vi "SADD.vi"(0 "TCP session out":refnum<k5>, 1 "Key":string, 5 "Members":string[](array[string]), 11 "error in":errorcluster) -> (4 "TCP session out":refnum<k5>, 6 "Data":T1, 15 "error out":errorcluster)   [LabVIEW 2023]
uses:
  SubVIs/Controls/redis-data.ctl
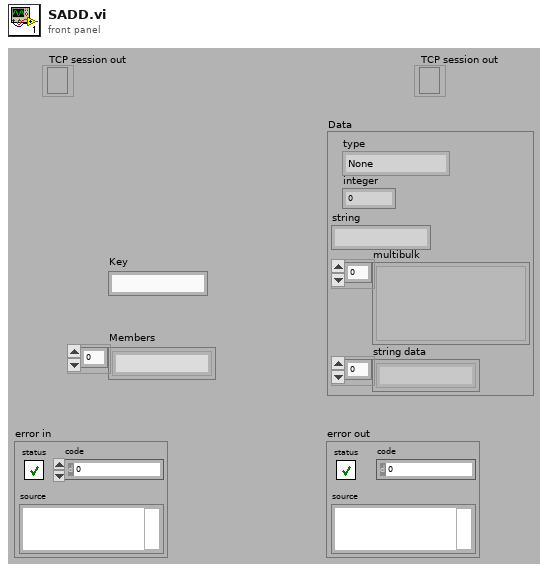
[diagram p1: front panel]
types:
  T1 = typedef "redis-data.ctl" = cluster{"type":enum16{"None", "Error", "Status", "Nil", "Integer", "String", "Multibulk"}, "integer":i64, "string":string, "multibulk":variant[], "string data":string[]}
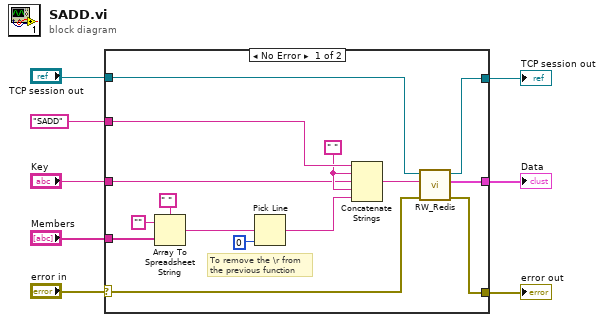
[diagram p0: block diagram]
diagram:
  n1 = case shown="No Error" "error in" {
    selector: "error in" -> [w21 w25]
    tunnel: "Members" -> [w14 _]
    tunnel: "SADD" -> [w23 _]
    tunnel: "TCP session out" -> [w10 w24]
    tunnel: [w20 w25] -> w6
    tunnel: [w19 _] -> w3
    tunnel: "Key" -> [w11 _]
    tunnel: [w9 w24] -> w1
    frame No Error {
      w13 = " "
      # "To remove the \\r from\nthe previous function"
      n2 = Array To Spreadsheet String(delimiter (Tab)=" ", array=w14, 3:"" ("format string")) -> (spreadsheet string=w17:string)
      n3 = Pick Line(multi-line string=w17, line index=0) -> (output string=w12:string)  [unwired: 1 in]
      n4 = Concatenate Strings(w23, w13, w11, w13, w12) -> (w22:string)
      n5 = call "RW_Redis.vi"("error in"=w21, "command"=w22, "TCP session in"=w10) -> ("error out"=w20:errorcluster, "Data"=w19:T1, "TCP session out"=w9:refnum<k5>)  [unwired: 6 in]
    }
    frame Error {
    }
  }
  "error out" <- w6
  "TCP session out" <- w1
  "Data" <- w3
